vi "Read Y.vi"(8 "error in (no error)":errorcluster, 11 "AssertEqualValue in":refnum<class "AssertAlmostEqualValue.lvclass">) -> (0 "error out":errorcluster, 2 "Y":ext, 3 "AssertEqualValue out":refnum<class "AssertAlmostEqualValue.lvclass">)   [LabVIEW 2021, in "Bananas.lvlib" / "AssertAlmostEqualValue.lvclass"]
uses:
  AssertAlmostEqualValue.lvclass
  AssertAlmostEqualValue.lvclass/AssertAlmostEqualValue.ctl
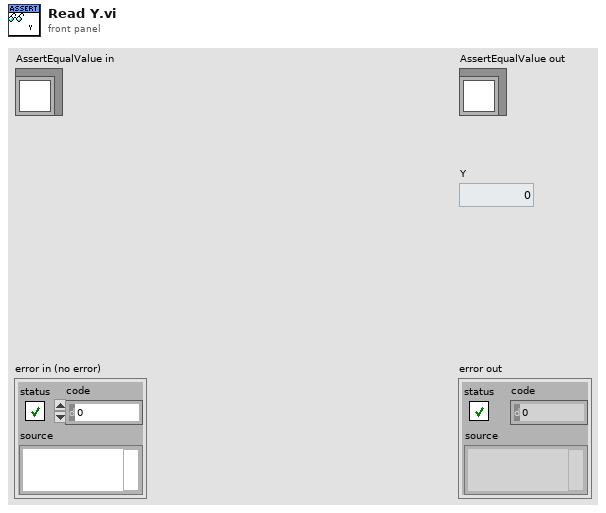
[diagram p1: front panel]
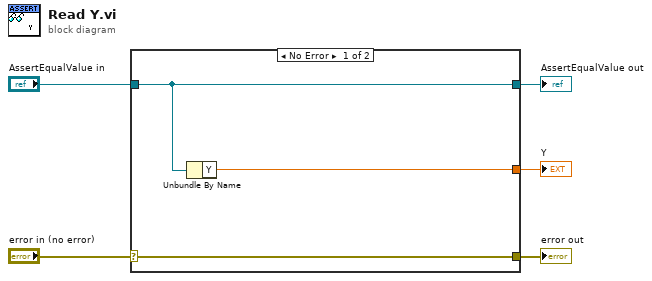
[diagram p0: block diagram]
diagram:
  n1 = case shown="No Error" "error in (no error)" {
    selector: "error in (no error)" -> [w8 w9]
    tunnel: [w8 w9] -> w4
    tunnel: [w7 w10] -> w2
    tunnel: "AssertEqualValue in" -> [w7 w10]
    tunnel: [w6 _] -> w1
    frame No Error {
      n2 = Unbundle By Name(w7) -> ("Y"=w6:ext)
    }
    frame Error {
    }
  }
  "error out" <- w4
  "AssertEqualValue out" <- w2
  "Y" <- w1
